vi "SetRef.vi"(8 "error in (no error)":errorcluster, 10 "Set External":bool, 11 "SpecA_MXA in":refnum<class "SpecA_MXA.lvclass">) -> (0 "error out":errorcluster, 3 "SpecA_MXA out":refnum<class "SpecA_MXA.lvclass">)   [LabVIEW 2014, in "SpecA_MXA.lvclass"]
uses:
  SpecA_MXA.lvclass
  SpecA_MXA.lvclass/SpecA_MXA.ctl
  <instrlib>/Agilent MXA Series/Agilent MXA Series.lvlib
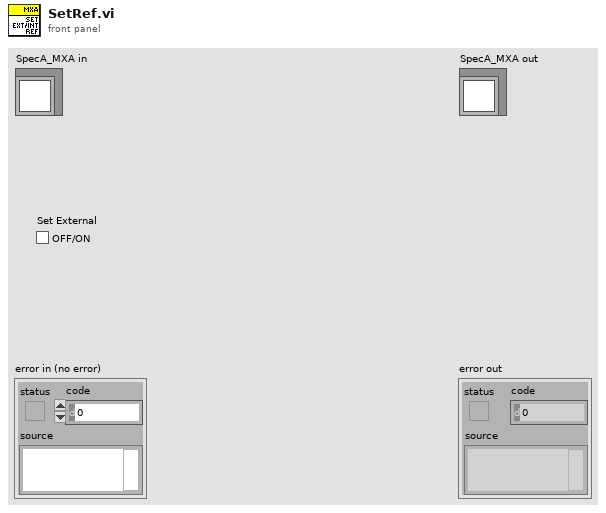
[diagram p1: front panel]
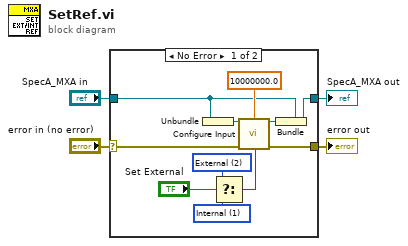
[diagram p0: block diagram]
diagram:
  n1 = case shown="No Error" "error in (no error)" {
    selector: "error in (no error)" -> [w10 w17]
    tunnel: [w9 w17] -> w4
    tunnel: [w5 w16] -> w3
    tunnel: "SpecA_MXA in" -> [w7 w16]
    frame No Error {
      w12 = 1 items=["Sense", "Internal", "External"] ("Frequency Reference In  (0:Sense)")
      w13 = 2 items=["Sense", "Internal", "External"] ("Frequency Reference In  (0:Sense)")
      n2 = Unbundle(w7) -> (w8:refnum<visa-resource-name>)
      n3 = Select(t=w13, s="Set External", f=w12) -> (s? t:f=w11:i32)
      n4 = call <instrlib>:"Configure Input.vi"("VISA resource name"=w8, "External Frequency (0 Hz)"=10000000.0, "error in (no error)"=w10, "Frequency Reference In  (0:Sense)"=w11) -> ("VISA resource name out"=w6:refnum<visa-resource-name>, "error out"=w9:errorcluster)  [unwired: 10 in]
      n5 = Bundle(cluster=w7, w6) -> (w5:refnum<class "SpecA_MXA.lvclass">)
    }
    frame Error {
    }
  }
  "error out" <- w4
  "SpecA_MXA out" <- w3
